vi "teleop drive filter.vi"(10 "input data":T1) -> (2 "output data":T1)   [LabVIEW 2013]
uses:
  dashboard/TeleopCmd.ctl
  CmdFlag.ctl
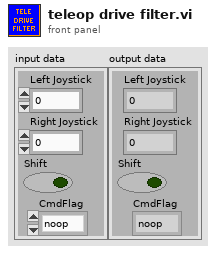
[diagram p1: front panel]
types:
  T1 = typedef "TeleopCmd.ctl" = cluster{"Left Joystick":dbl, "Right Joystick":dbl, "Shift":bool, "CmdFlag":T2}
  T2 = typedef "CmdFlag.ctl" = enum16{"noop", "suspend", "resume"}
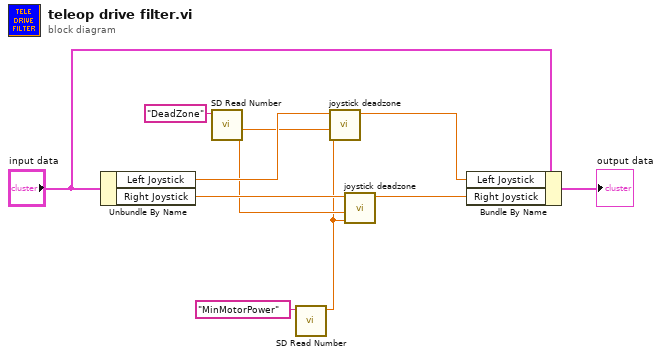
[diagram p0: block diagram]
diagram:
  n1 = Unbundle By Name("input data") -> ("Left Joystick"=w8:dbl, "Right Joystick"=w6:dbl)
  n2 = call <vilib>:"SD Read Number.vi"("Name"="DeadZone") -> ("Numeric"=w2:dbl)  [unwired: 8 in, 2 out]
  n3 = call <vilib>:"SD Read Number.vi"("Name"="MinMotorPower") -> ("Numeric"=w1:dbl)  [unwired: 8 in, 2 out]
  n4 = call "joystick deadzone.vi"("minpower"=w1, "deadzone"=w2, "joystick"=w8) -> ("joyout"=w7:dbl)  [unwired: 8 in]
  n5 = call "joystick deadzone.vi"("minpower"=w1, "deadzone"=w2, "joystick"=w6) -> ("joyout"=w5:dbl)  [unwired: 8 in]
  n6 = Bundle By Name(cluster="input data", "Left Joystick"=w7, "Right Joystick"=w5) -> (→"output data":T1)
